vi "HostVI.vi"() -> ()   [LabVIEW 2014]
uses:
  Controls/State.ctl
  <vilib>/rvi/interface/RandomDataEmulation/nirviRandomDataOpen.vi
  <vilib>/rvi/interface/common/niFpgaCacheSessionInfoDynamic.vi
  <vilib>/FPGAPlugInAG/Dynamic/niLvFpga_Close_Dynamic.vi
  <vilib>/Utility/error.llb/Error Cluster From Error Code.vi
  <vilib>/rvi/errors/niLvFpgaAdjustHostInterfaceError.vi
  <vilib>/rvi/interface/nirviOpenFPGA/nirviOpenFPGA.xnode
  FPGA_VI.vi
  <vilib>/rvi/interface/nirviCloseFPGA/nirviCloseFPGA.xnode
  <vilib>/rvi/interface/nirviReadWriteControl/nirviReadWriteControl.xnode
  <vilib>/rvi/interface/nirviMethod/nirviMethod.xnode
  NiFpgaLv.dll
  <vilib>/rvi/interface/Simulation/niFpgaSimulationCallBeginRW.vi
  <vilib>/FPGAPlugInAG/Dynamic/niLvFpga_ReadFifo_Dynamic.vi
  <vilib>/rvi/errors/niLvFpgaMergeErrorWithErrorCode.vi
panel:
  in  "stop":bool
  out "Channels 12-15":dbl[][](graph)
  out "Channels 8-11":dbl[][](graph)
  out "Channels 4-7":dbl[][](graph)
  out "Channels 0-3":dbl[][](graph)
  out "error out":errorcluster
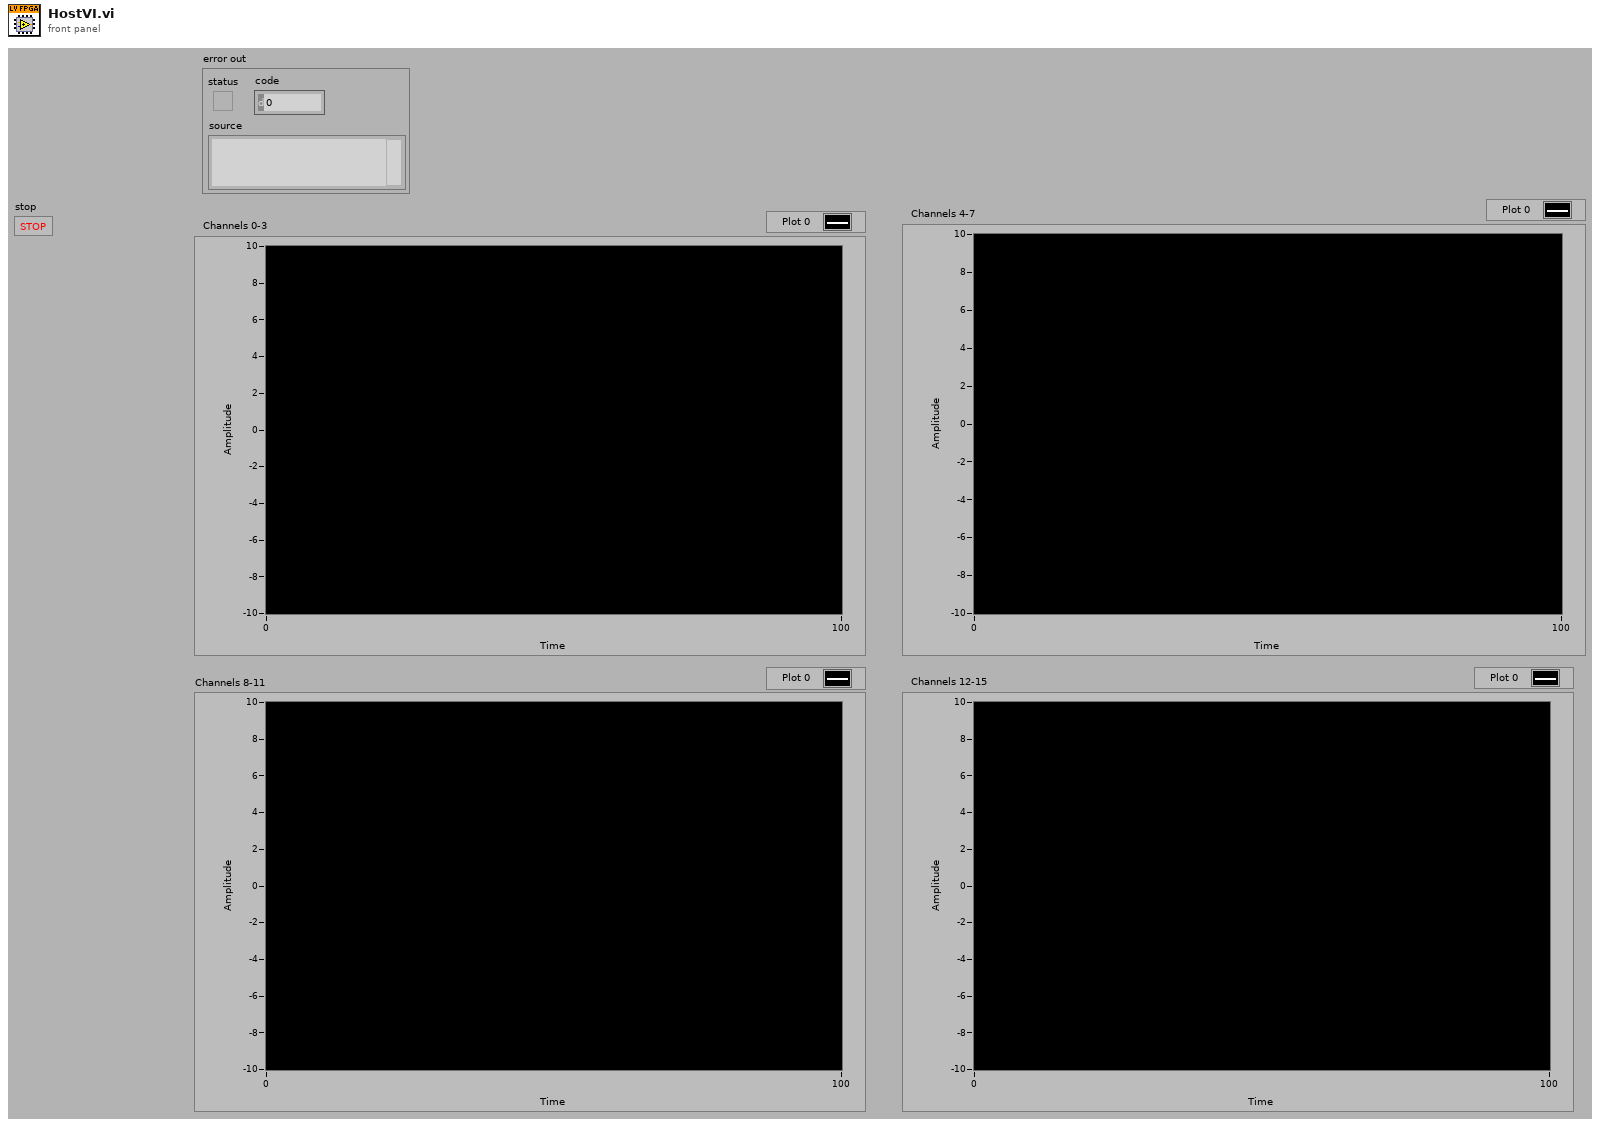
[diagram p1: front panel]
types:
  T1 = typedef "State.ctl" = enum16{"Trigger", "Fetch Data DRAM 0", "Fetch Data DRAM 1", "Graph Data", "Shut Down"}
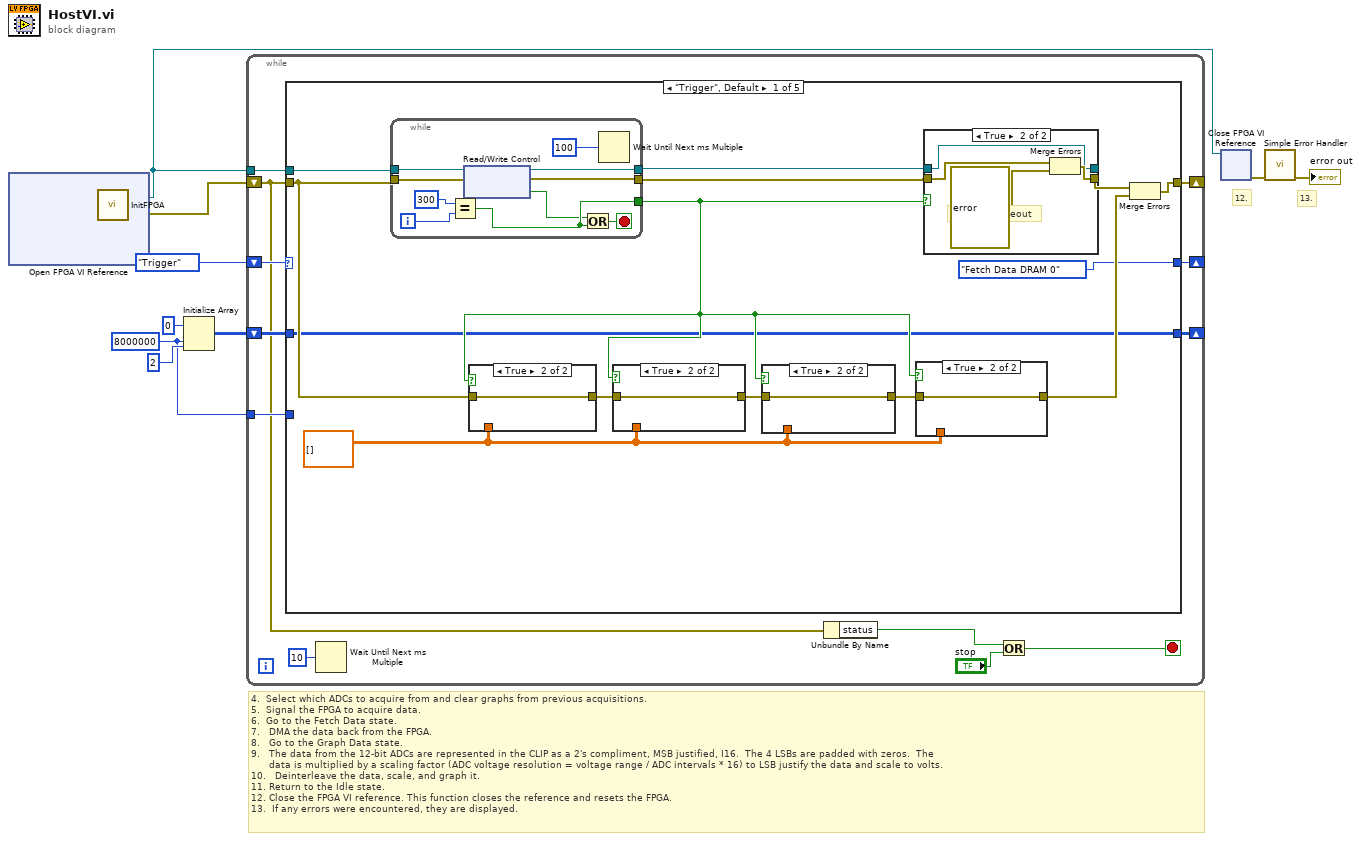
[diagram p0: block diagram]
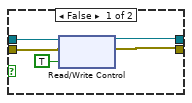
[diagram p2: hidden frame]
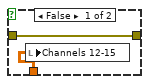
[diagram p3: hidden frame]
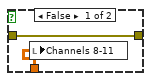
[diagram p4: hidden frame]
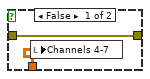
[diagram p5: hidden frame]
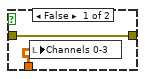
[diagram p6: hidden frame]
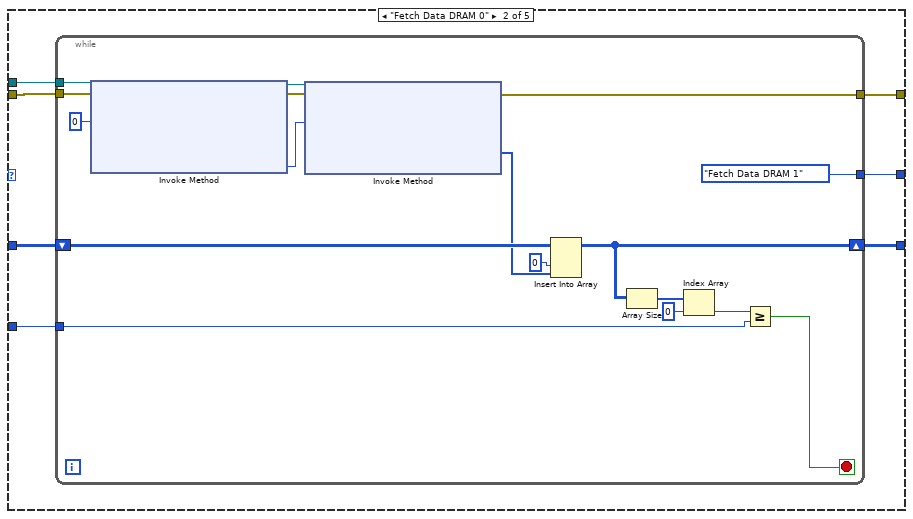
[diagram p7: hidden frame]
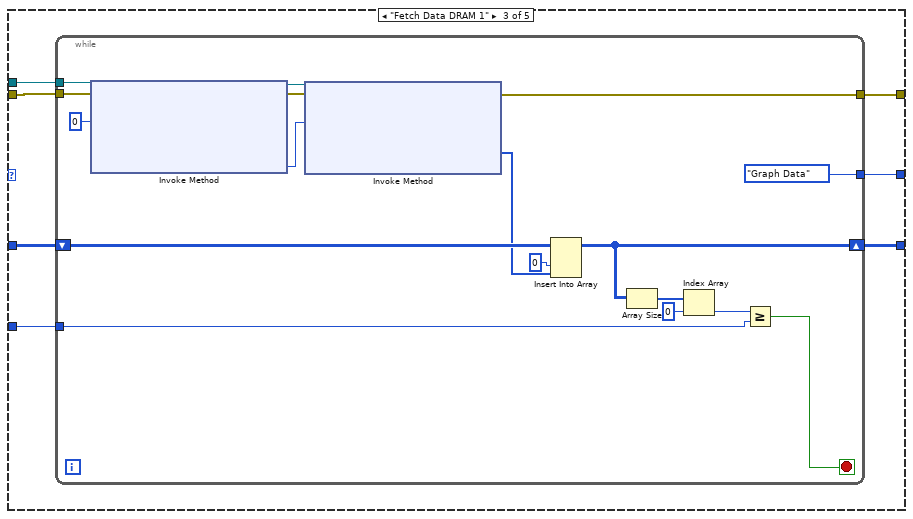
[diagram p8: hidden frame]
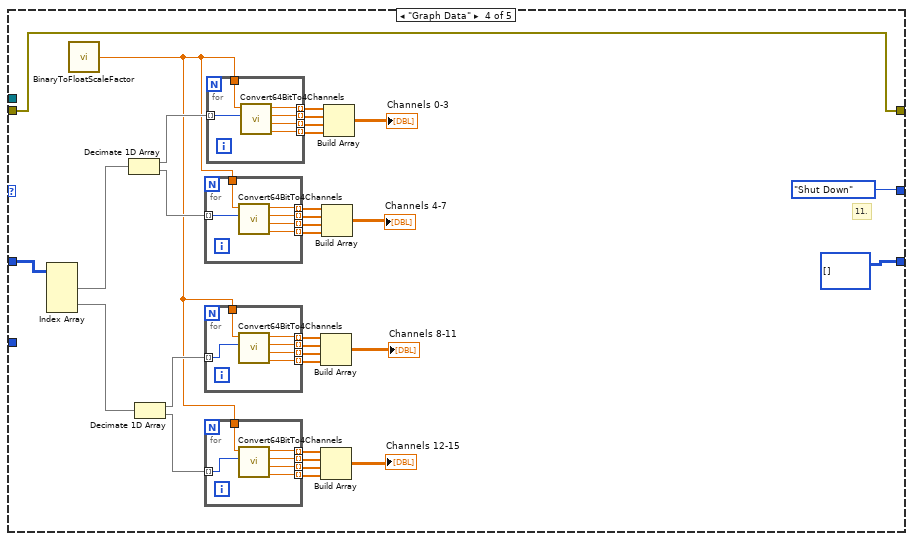
[diagram p9: hidden frame]
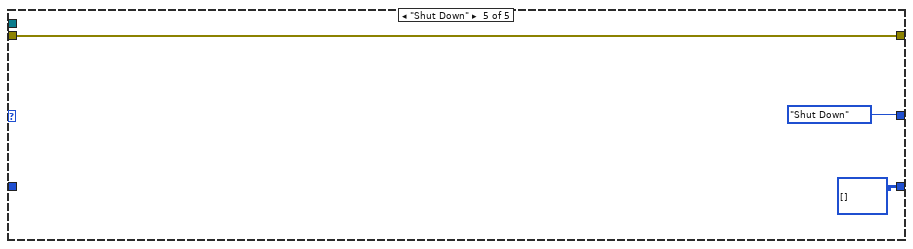
[diagram p10: hidden frame]
diagram:
  w2 = 8000000 ("dimension size")
  # "13."
  # "12."
  # "4.  Select which ADCs to acquire from and clear graphs from previous acquisitions.\n5.  Signal the FPGA to acquire data.\n6.  Go to the Fetch Data state.\n7.   DMA the data back from the FPGA.\n8.   Go to the Graph Data state.\n9.   The data from the 12-bit ADCs are represented in the CLIP as a 2's compliment, MSB justified, I16.  The 4 LSBs are padded with zeros.  The \n      data is multiplied by a scaling factor (ADC voltage resolution = voltage range / ADC intervals * 16) to LSB justify the data and scale to volts.\n10.   Deinterleave the data, scale, and graph it.\n11. Return to the Idle state.\n12. Close the FPGA VI reference. This function closes the reference and resets the FPGA.\n13.  If any errors were encountered, they are displayed."
  n1 = xnode "Open FPGA VI Reference"() -> ("FPGA VI Reference Out"=w9:refnum<k20>, "error out"=w7:errorcluster)  [unwired: 2 in]
  n2 = call "InitFPGA.vi"("error in"=w7, "FPGA VI Reference In"=w9) -> ("error out"=w6:errorcluster, "FPGA VI Reference Out"=w8:refnum<k20>)
  n3 = Initialize Array(u64 0 ("element"), w2, 2 ("dimension size")) -> (w3:u64[][])
  n4 = while {
    tunnel: w8 -> [w22]
    shift-right: [w19] -> _
    shift-left: w6 -> [w13]
    shift-right: [w16] -> _
    shift-left: w3 -> [w18]
    tunnel: w2 -> [w17]
    shift-right: [w14] -> _
    shift-left: State."Trigger" -> [w15]
    stop <- w20 stop-if-true
    n5 = case shown="\"Trigger\", Default" w15 {
      tunnel: w22 -> [w30 w75 w99 _ _]
      tunnel: w13 -> [w29 w74 w98 w119 w174]
      tunnel: [w25 w73 w97 w119 w174] -> w19
      tunnel: w18 -> [w24 w72 w96 w147 _]
      tunnel: w17 -> [_ w71 w95 _ _]
      tunnel: [w24 w70 w94 u64[][] [] u64[][] []] -> w16
      tunnel: [State."Fetch Data DRAM 0" w69 w93 State."Shut Down" State."Shut Down"] -> w14
      frame "Trigger", Default {
        w36 = dbl[][] [] ("ADC A Graph")
        n6 = while {
          tunnel: w30 -> [w56]
          tunnel: [w52] -> w31
          tunnel: [w51] -> w28
          tunnel: [w49] -> w26
          tunnel: w29 -> [w47]
          i -> [w54]
          stop <- w50 stop-if-true
          n7 = Equal?(x=300, y=w54) -> (x = y?=w49:bool)
          n8 = xnode "Read/Write Control"("FPGA VI Reference In"=w56, "error in"=w47) -> ("FPGA VI Reference Out"=w52:refnum<k20>, "error out"=w51:errorcluster, "Init Done"=w48:bool)
          n9 = Or(x=w48, y=w49) -> (x .or. y?=w50:bool)
          n10 = Wait Until Next ms Multiple(millisecond multiple=u32 100) -> ()  [unwired: 1 out]
        }
        n11 = case shown="True" w26 {
          tunnel: w29 -> [w66 w68]
          tunnel: w36 -> [w67 _]
          tunnel: [w66 w68] -> w35
          frame False {
            n12 = local write "Channels 0-3"(w67) -> ()
          }
          frame True {
          }
        }
        n13 = case shown="True" w26 {
          tunnel: w36 -> [w64 _]
          tunnel: w35 -> [w63 w65]
          tunnel: [w63 w65] -> w34
          frame False {
            n14 = local write "Channels 4-7"(w64) -> ()
          }
          frame True {
          }
        }
        n15 = case shown="True" w26 {
          tunnel: w36 -> [w61 _]
          tunnel: w34 -> [w60 w62]
          tunnel: [w60 w62] -> w33
          frame False {
            n16 = local write "Channels 8-11"(w61) -> ()
          }
          frame True {
          }
        }
        n17 = case shown="True" w26 {
          tunnel: [w57 w59] -> w37
          tunnel: w36 -> [w58 _]
          tunnel: w33 -> [w57 w59]
          frame False {
            n18 = local write "Channels 12-15"(w58) -> ()
          }
          frame True {
          }
        }
        n19 = case shown="True" w26 {
          tunnel: [w40 w44] -> _
          tunnel: w31 -> [w42 w44]
          tunnel: w28 -> [w41 w43]
          tunnel: [w39 w46] -> w32
          frame False {
            n20 = xnode "Read/Write Control"("FPGA VI Reference In"=w42, "error in"=w41, "Trigger"=TRUE) -> ("FPGA VI Reference Out"=w40:refnum<k20>, "error out"=w39:errorcluster)
          }
          frame True {
            # "InitDone timeout"
            n21 = Merge Errors(w43, errorcluster {"status"=TRUE, "code"=-1, "source"="The IO Module CLIP was not ready. If you are using any external clocks, make sure they are connected and within the supported specifications."} ("error in")) -> (w46:errorcluster)
          }
        }
        n22 = Merge Errors(w32, w37) -> (w25:errorcluster)
      }
      frame "Fetch Data DRAM 0" {
        n23 = while {
          tunnel: w75 -> [w92]
          tunnel: w74 -> [w89]
          tunnel: [w88] -> w73
          shift-right: [w82] -> w70
          shift-left: w72 -> [w85]
          tunnel: w71 -> [w77]
          tunnel: [State."Fetch Data DRAM 1"] -> w69
          stop <- w78 stop-if-true
          n24 = xnode "Invoke Method"("FPGA VI Reference In"=w92, "error in"=w89, "Number of Elements"=u32 0) -> ("FPGA VI Reference Out"=w86:refnum<k20>, "error out"=w87:errorcluster, "Elements Remaining"=w91:u32)  [unwired: 1 in, 1 out]
          n25 = xnode "Invoke Method"("FPGA VI Reference In"=w86, "error in"=w87, "Number of Elements"=w91) -> ("error out"=w88:errorcluster, "Data"=w84:u64[])  [unwired: 1 in, 2 out]
          n26 = Insert Into Array(array=w85, index (col)=0 ("disabled index (col)"), new element=w84) -> (w82:u64[][])  [unwired: 1 in]
          n27 = Array Size(array=w82) -> (size(s)=w81:i32[])
          n28 = Index Array(array=w81, index=0) -> (element=w79:i32)
          n29 = Greater Or Equal?(x=w79, y=w77) -> (x >= y?=w78:bool)
        }
      }
      frame "Fetch Data DRAM 1" {
        n30 = while {
          tunnel: w99 -> [w116]
          tunnel: w98 -> [w113]
          tunnel: [w112] -> w97
          shift-right: [w106] -> w94
          shift-left: w96 -> [w109]
          tunnel: w95 -> [w101]
          tunnel: [State."Graph Data"] -> w93
          stop <- w102 stop-if-true
          n31 = xnode "Invoke Method"("FPGA VI Reference In"=w116, "error in"=w113, "Number of Elements"=u32 0) -> ("FPGA VI Reference Out"=w110:refnum<k20>, "error out"=w111:errorcluster, "Elements Remaining"=w115:u32)  [unwired: 1 in, 1 out]
          n32 = xnode "Invoke Method"("FPGA VI Reference In"=w110, "error in"=w111, "Number of Elements"=w115) -> ("error out"=w112:errorcluster, "Data"=w108:u64[])  [unwired: 1 in, 2 out]
          n33 = Insert Into Array(array=w109, index (col)=0 ("disabled index (col)"), new element=w108) -> (w106:u64[][])  [unwired: 1 in]
          n34 = Array Size(array=w106) -> (size(s)=w105:i32[])
          n35 = Index Array(array=w105, index=0) -> (element=w103:i32)
          n36 = Greater Or Equal?(x=w103, y=w101) -> (x >= y?=w102:bool)
        }
      }
      frame "Graph Data" {
        # "11."
        n37 = Index Array(array=w147) -> (element #1=w134:u64[], element #2=w127:u64[])  [unwired: 4 in]
        n38 = call "BinaryToFloatScaleFactor.vi"() -> ("Scale Factor"=w124:dbl)  [unwired: 2 in]
        n39 = Decimate 1D Array(w134) -> (w133:u64[], w132:u64[])
        n40 = Decimate 1D Array(w127) -> (w126:u64[], w125:u64[])
        n41 = for {
          tunnel: [w159] -> w138 mode=indexing
          tunnel: w124 -> [w158]
          tunnel: [w157] -> w137 mode=indexing
          tunnel: [w156] -> w136 mode=indexing
          tunnel: [w155] -> w135 mode=indexing
          tunnel: w132 -> [w154] mode=indexing
          n42 = call "Convert64BitTo4Channels.vi"("64 Bit Int"=w154, "Scale Factor"=w158) -> ("Channel 3"=w155:dbl, "Channel 2"=w156:dbl, "Channel 1"=w157:dbl, "Channel 0"=w159:dbl)  [unwired: 6 in]
        }
        n43 = for {
          tunnel: w126 -> [w165] mode=indexing
          tunnel: [w164] -> w142 mode=indexing
          tunnel: w124 -> [w163]
          tunnel: [w162] -> w141 mode=indexing
          tunnel: [w161] -> w139 mode=indexing
          tunnel: [w160] -> w140 mode=indexing
          n44 = call "Convert64BitTo4Channels.vi"("64 Bit Int"=w165, "Scale Factor"=w163) -> ("Channel 3"=w160:dbl, "Channel 2"=w161:dbl, "Channel 1"=w162:dbl, "Channel 0"=w164:dbl)  [unwired: 6 in]
        }
        n45 = for {
          tunnel: w125 -> [w149] mode=indexing
          tunnel: [w153] -> w131 mode=indexing
          tunnel: [w152] -> w130 mode=indexing
          tunnel: [w151] -> w128 mode=indexing
          tunnel: [w150] -> w129 mode=indexing
          tunnel: w124 -> [w148]
          n46 = call "Convert64BitTo4Channels.vi"("64 Bit Int"=w149, "Scale Factor"=w148) -> ("Channel 3"=w150:dbl, "Channel 2"=w151:dbl, "Channel 1"=w152:dbl, "Channel 0"=w153:dbl)  [unwired: 6 in]
        }
        n47 = for {
          tunnel: [w171] -> w146 mode=indexing
          tunnel: w124 -> [w170]
          tunnel: [w169] -> w145 mode=indexing
          tunnel: [w168] -> w144 mode=indexing
          tunnel: [w167] -> w143 mode=indexing
          tunnel: w133 -> [w166] mode=indexing
          n48 = call "Convert64BitTo4Channels.vi"("64 Bit Int"=w166, "Scale Factor"=w170) -> ("Channel 3"=w167:dbl, "Channel 2"=w168:dbl, "Channel 1"=w169:dbl, "Channel 0"=w171:dbl)  [unwired: 6 in]
        }
        n49 = Build Array(w142, w141, w139, w140) -> (→"Channels 8-11":dbl[][])
        n50 = Build Array(w131, w130, w128, w129) -> (→"Channels 12-15":dbl[][])
        n51 = Build Array(w138, w137, w136, w135) -> (→"Channels 4-7":dbl[][])
        n52 = Build Array(w146, w145, w144, w143) -> (→"Channels 0-3":dbl[][])
      }
      frame "Shut Down" {
      }
    }
    n53 = Wait Until Next ms Multiple(millisecond multiple=u32 10) -> ()  [unwired: 1 out]
    n54 = Unbundle By Name(w13) -> ("status"=w21:bool)
    n55 = Or(x=w21, y="stop") -> (x .or. y?=w20:bool)
  }
  n56 = xnode "Close FPGA VI Reference"("FPGA VI Reference In"=w8) -> ("error out"=w11:errorcluster)  [unwired: 1 in]
  n57 = call <vilib>:"Simple Error Handler.vi"("error in (no error)"=w11) -> ("error out"=→"error out":errorcluster)  [unwired: 1 in, 7 out]
